vi "CDMA_TxRFloopback.vi"(6 "xsrpip":string, 7 "pcip":string, 8 "error in (no error)":errorcluster caption="错误输入（无错误）", 9 "system_type":dbl, 10 "tx_data":cdb[](array[numeric]), 11 "Path In":path) -> (0 "error out":errorcluster caption="错误输出", 3 "Path Out":path)   [LabVIEW 2015]
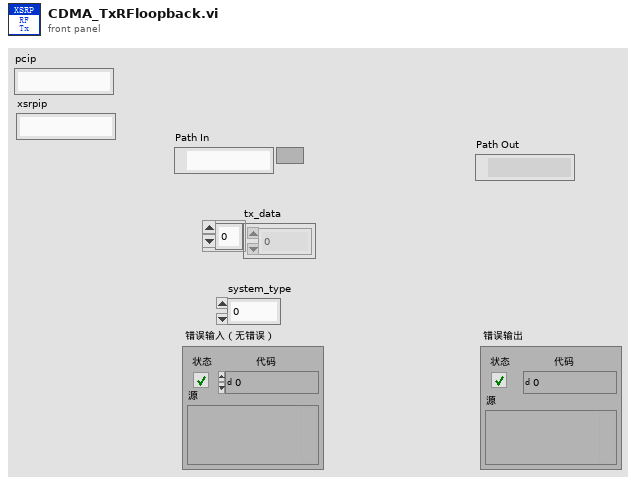
[diagram p1: front panel]
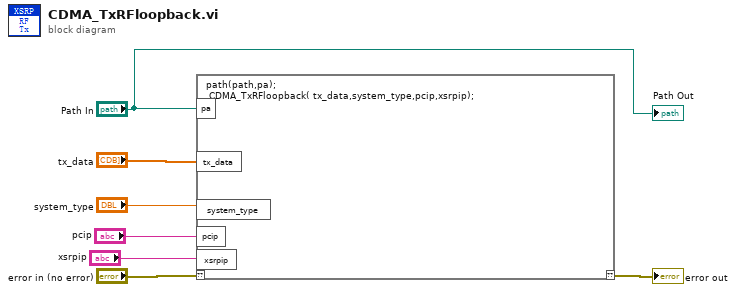
[diagram p0: block diagram]
diagram:
  n1 = script code="path(path,pa);\n CDMA_TxRFloopback( tx_data,system_type,pcip,xsrpip);"("??"="error in (no error)", "pa"="Path In", "tx_data"="tx_data", "system_type"="system_type", "pcip"="pcip", "xsrpip"="xsrpip") -> ("??"=→"error out":errorcluster)
  "Path Out" <- "Path In"
